vi "InitTH260_AnyThread.vi"(8 "error in (no error)":errorcluster, 9 "MeasMode":T3 items=["Histo"=0, "T2"=2, "T3"=3, "Conti"=8], 10 "TimingMode":T1 items=["Hires", "Lowres"], 11 "Library Version":string="3.1") -> (0 "error out":errorcluster, 2 "Init Info":T2, 3 "DevIdx":i32)   [LabVIEW 2017]
uses:
  TH260_MeasMode.ctl
  TH260_InitInfo.ctl
  TH260_TimingMode.ctl
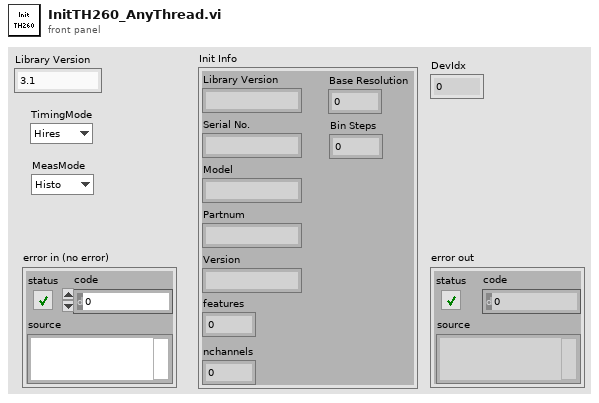
[diagram p1: front panel]
types:
  T1 = typedef "TH260_TimingMode.ctl" = i32
  T2 = typedef "TH260_InitInfo.ctl" = cluster{"Library Version":string, "Serial No.":string, "Model":string, "Partnum":string, "Version":string, "features":i32, "nchannels":i32, "Base Resolution":dbl, "Bin Steps":i32}
  T3 = typedef "TH260_MeasMode.ctl" = i32
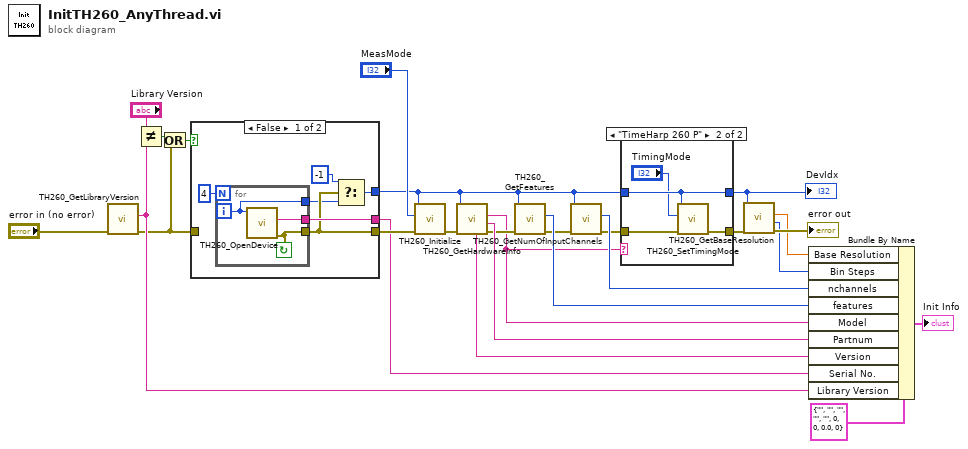
[diagram p0: block diagram]
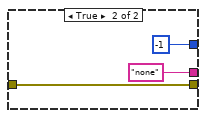
[diagram p3: hidden frame]
diagram:
  n1 = call "TH260_GetLibraryVersion.vi"("error in (no error)"="error in (no error)") -> ("error out"=w7:errorcluster, "Version"=w15:string)  [unwired: 8 in, 1 out]
  n2 = Not Equal?(x="Library Version", y=w15) -> (x != y?=w25:bool)
  n3 = Or(x=w25, y=w7) -> (x .or. y?=w24:bool)
  n4 = case shown="False" w24 {
    tunnel: [w28 -1 ("return type")] -> w4
    tunnel: [w31 "none" ("serial")] -> w17
    tunnel: [w30 w36] -> w23
    tunnel: w7 -> [_ w36]
    frame False {
      n5 = for {
        N: 4 -> [_]
        tunnel: [w34] -> w30
        tunnel: [w33] -> w31
        tunnel: [w35] -> w29
        i -> [w35]
        stop <- w34 continue-if-true
        n6 = call "TH260_OpenDevice.vi"("devidx"=w35) -> ("error out"=w34:errorcluster, "serial"=w33:string)  [unwired: 8 in, 1 out]
      }
      n7 = Select(t=-1, s=w30, f=w29) -> (s? t:f=w28:i32)
    }
    frame True {
    }
  }
  n8 = call "TH260_Initialize.vi"("error in (no error)"=w23, "mode"="MeasMode", "devidx"=w4) -> ("error out"=w21:errorcluster)  [unwired: 7 in, 1 out]
  n9 = call "TH260_GetHardwareInfo.vi"("error in (no error)"=w21, "devidx"=w4) -> ("error out"=w13:errorcluster, "Partnum"=w20:string, "Model"=w5:string, "Version"=w19:string)  [unwired: 5 in, 1 out]
  n10 = call "TH260_GetFeatures.vi"("error in (no error)"=w13, "devidx"=w4) -> ("error out"=w6:errorcluster, "features"=w18:i32)  [unwired: 7 in, 1 out]
  n11 = call "TH260_GetNumOfInputChannels.vi"("error in (no error)"=w6, "devidx"=w4) -> ("error out"=w3:errorcluster, "nchannels"=w12:i32)  [unwired: 7 in, 1 out]
  n12 = case shown="\"TimeHarp 260 P\"" w5 {
    tunnel: w4 -> [w39 w42]
    tunnel: w3 -> [w40 w44]
    tunnel: [w40 w43] -> w2
    tunnel: [w39 w42] -> w1
    frame Default {
    }
    frame "TimeHarp 260 P" {
      n13 = call "TH260_SetTimingMode.vi"("error in (no error)"=w44, "mode"="TimingMode", "devidx"=w42) -> ("error out"=w43:errorcluster)  [unwired: 7 in, 1 out]
    }
  }
  "DevIdx" <- w1
  n14 = call "TH260_GetBaseResolution.vi"("error in (no error)"=w2, "devidx"=w1) -> ("error out"=→"error out":errorcluster, "binsteps"=w10:i32, "resolution"=w9:dbl)  [unwired: 6 in, 1 out]
  n15 = Bundle By Name(cluster=T2 {"Library Version"="", "Serial No."="", "Model"="", "Partnum"="", "Version"="", "features"=0, "nchannels"=0, "Base Resolution"=0.0, "Bin Steps"=0} ("Init"), "Base Resolution"=w9, "Bin Steps"=w10, "nchannels"=w12, "features"=w18, "Model"=w5, "Partnum"=w20, "Version"=w19, "Serial No."=w17, "Library Version"=w15) -> (→"Init Info":T2)
